vi "Init Line.vi"(7 "Color (RGB black)":refnum<class "Color.lvclass">=refnum, 8 "error in (no error)":errorcluster, 9 "end point (0,0)":cluster{"x":i16, "y":i16}, 10 "start point (0,0)":cluster{"x":i16, "y":i16}, 11 "Line in":refnum<class "Line.lvclass">) -> (0 "error out":errorcluster, 3 "Line out":refnum<class "Line.lvclass">)   [LabVIEW 2018, in "Line.lvclass"]
doc: "Initialize a line"
uses:
  Line.lvclass
  Color/Color.lvclass
  RGB Color/RGB Color.lvclass
  Graphics Object/Graphics Object.lvclass
panel:
  # "expressionflow.com"
  # "Copyright (c) 2008 Tomi Maila. All rights reserved."
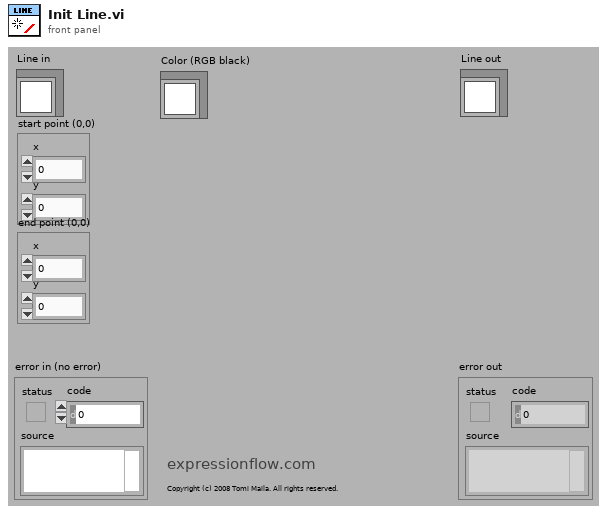
[diagram p1: front panel]
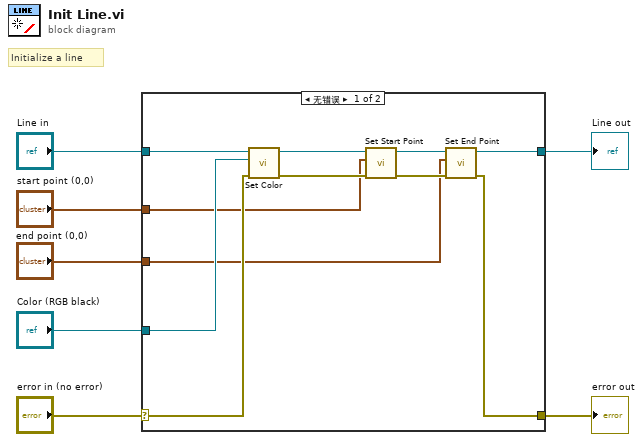
[diagram p0: block diagram]
diagram:
  # "Initialize a line"
  n1 = case shown="无错误" "error in (no error)" {
    selector: "error in (no error)" -> [w17 w20]
    tunnel: [w11 w20] -> w6
    tunnel: [w8 w19] -> w4
    tunnel: "Line in" -> [w18 w19]
    tunnel: "start point (0,0)" -> [w10 _]
    tunnel: "end point (0,0)" -> [w9 _]
    tunnel: "Color (RGB black)" -> [w16 _]
    frame No Error {
      n2 = call-dynamic "Set Color.vi"("error in (no error)"=w17, "Color (RGB black)"=w16, "Geometric Object.lvclass in"=w18) -> ("error out"=w12:errorcluster, "Geometric Object.lvclass out"=w15:refnum<class "Line.lvclass">)  [unwired: 7 in]
      n3 = call "Set Start Point.vi"("error in (no error)"=w12, "start point (0,0)"=w10, "Graphics Object.lvclass in"=w15) -> ("error out"=w13:errorcluster, "Graphics Object.lvclass out"=w14:refnum<class "Line.lvclass">)  [unwired: 7 in]
      n4 = call "Set End Point.vi"("error in (no error)"=w13, "end point (0,0)"=w9, "Graphics Object.lvclass in"=w14) -> ("error out"=w11:errorcluster, "Graphics Object.lvclass out"=w8:refnum<class "Line.lvclass">)  [unwired: 7 in]
    }
    frame Error {
    }
  }
  "error out" <- w6
  "Line out" <- w4
